vi "Read Async Queue Timeout.vi"(8 "error in":errorcluster, 11 "Module Editor Node in":refnum<class "module editor node.lvclass">) -> (0 "error out":errorcluster, 2 "Queue Timeout":i32, 3 "Module Editor Node out":refnum<class "module editor node.lvclass">)   [LabVIEW 2013, in "PL Framework Configuration Tool.lvlib" / "module editor node.lvclass"]
uses:
  module editor node.lvclass
  module editor node.lvclass/module editor node.ctl
  asynchronous execution module/configuration/asynchronous execution module configuration.lvclass/asynchronous execution module configuration.ctl
  asynchronous execution module/configuration/asynchronous execution module configuration.lvclass
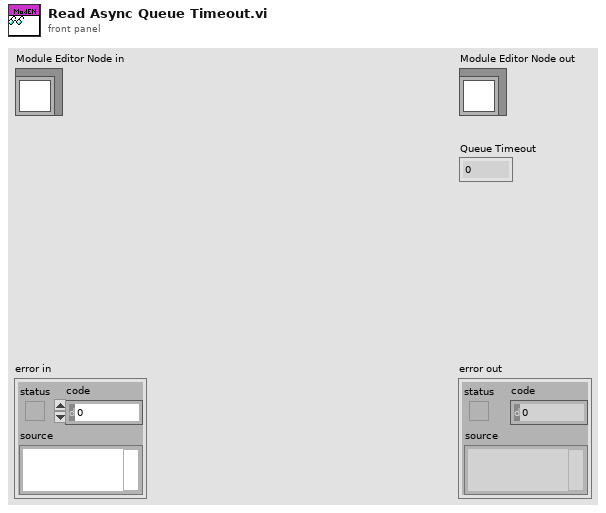
[diagram p1: front panel]
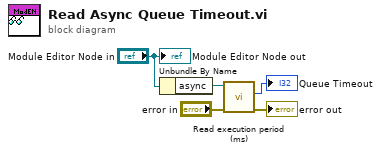
[diagram p0: block diagram]
diagram:
  n1 = Unbundle By Name("Module Editor Node in") -> ("async"=w4:refnum<class "asynchronous execution module configuration.lvclass">)
  n2 = call "Read execution period (ms).vi"("error in"="error in", "Asynchronous Component Configuration in"=w4) -> ("error out"=→"error out":errorcluster, "execution period (ms)"=→"Queue Timeout":i32)  [unwired: 7 in, 1 out]
  "Module Editor Node out" <- "Module Editor Node in"
